vi "ServerFirst.vi"(8 "error in (no error)":errorcluster, 10 "Challenge data in":T1, 11 "WampScramAuthenticator in":refnum<class "WampScramAuthenticator.lvclass">) -> (0 "error out":errorcluster, 1 "ServerFirst":string, 2 "Challenge data out":T1, 3 "WampScramAuthenticator out":refnum<class "WampScramAuthenticator.lvclass">)   [LabVIEW 2020, in "wamplv.lvlib" / "WampScramAuthenticator.lvclass"]
uses:
  WampScramAuthenticator.lvclass
  TypeDefs/Challenge data.ctl
  TypeDefs/HMAC parameters.ctl
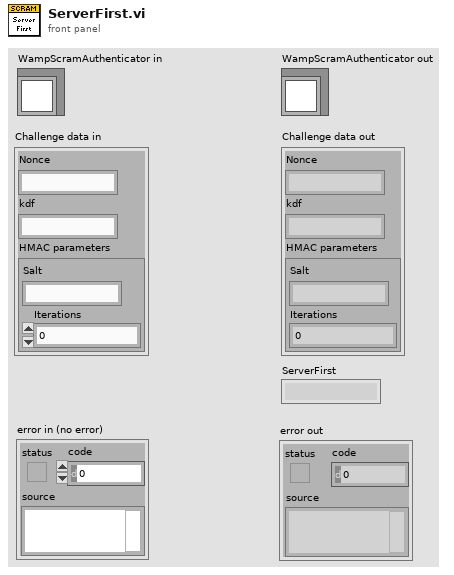
[diagram p1: front panel]
types:
  T1 = typedef "wamplv.lvlib/WampScramAuthenticator.lvclass/Challenge data.ctl" = cluster{"Nonce":string, "kdf":string, "HMAC parameters":T2}
  T2 = typedef "wamplv.lvlib/WampScramAuthenticator.lvclass/HMAC parameters.ctl" = cluster{"Salt":string, "Iterations":i32}
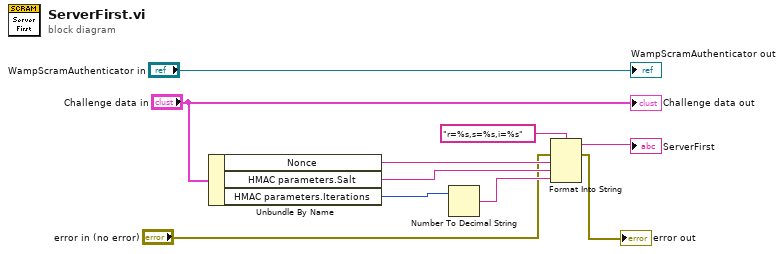
[diagram p0: block diagram]
diagram:
  n1 = Unbundle By Name("Challenge data in") -> ("Nonce"=w8:string, "HMAC parameters.Salt"=w7:string, "HMAC parameters.Iterations"=w6:i32)
  n2 = Number To Decimal String(number=w6) -> (decimal integer string=w5:string)  [unwired: 1 in]
  n3 = Format Into String(format string="r=%s,s=%s,i=%s", error in="error in (no error)", w8, w7, w5) -> (resulting string=→"ServerFirst":string, error out=→"error out":errorcluster)  [unwired: 1 in]
  "WampScramAuthenticator out" <- "WampScramAuthenticator in"
  "Challenge data out" <- "Challenge data in"
